vi "ExportDependencyItemRuleContent.vi"(8 "error in (no error)":errorcluster, 10 "IDependencyItemRule in":refnum<class "IDependencyItemRule.lvclass">, 11 "CGrapherDGML in":refnum<class "CGrapherDGML.lvclass">) -> (0 "error out":errorcluster, 1 "Links":T1, 2 "Nodes":T1, 3 "CGrapherDGML":refnum<class "CGrapherDGML.lvclass">)   [LabVIEW 2020, in "DefaultExtensions.lvlib" / "CGrapherDGML.lvclass"]
uses:
  CGrapherDGML.lvclass
  obj/Addons/LabVIEWObjectInterfaces.lvlibp/LabVIEWObjectInterfaces/IDependencyItemRule/IDependencyItemRule.lvclass
  E:/Repos/LVDependencyInspector/obj/Addons/LabVIEWObjectInterfaces.lvlibp/LabVIEWObjectInterfaces/ILabVIEWItem/ILabVIEWItem.lvclass
  obj/Addons/LabVIEWItem.lvlibp/LabVIEWItem/CLabVIEWItem/ConnectionSet.ctl
  CGrapherDGML.lvclass/CGrapherDGML.ctl
  84b6f64b-e02b-4565-8a95-97306d3fff3e.vi
  5ae37459-432d-44eb-8d2b-a2ae9b2d80af.vi
  0dec89c7-531e-457a-9eb0-0c91c63ee5dd.vi
  obj/Addons/LabVIEWItem.lvlibp/LabVIEWItem/CLabVIEWItem/CLabVIEWItem.lvclass
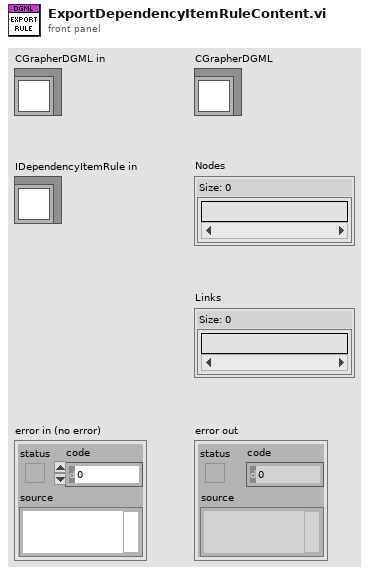
[diagram p1: front panel]
types:
  T1 = typedef "LabVIEWItem.lvlibp/CLabVIEWItem.lvclass/ConnectionSet.ctl" = set{string}
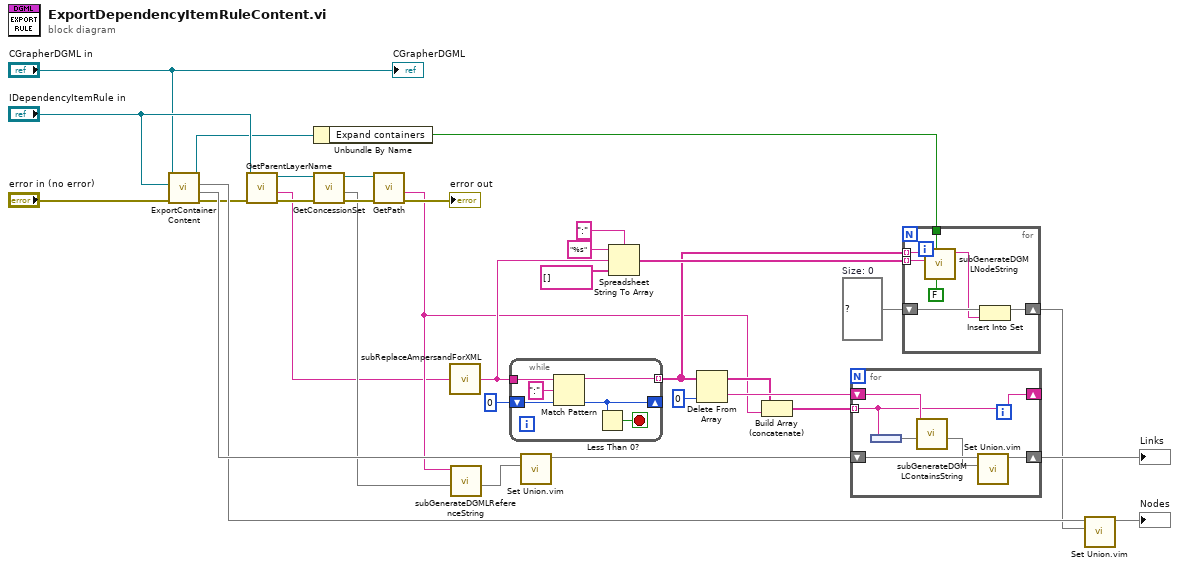
[diagram p0: block diagram]
diagram:
  w20 = set{string} {}  # Size: 0
  n1 = call-dynamic "ExportContainerContent.vi"("error in (no error)"="error in (no error)", "ILabVIEWItem in"="IDependencyItemRule in", "CGrapherDGML in"="CGrapherDGML in") -> ("error out"=w8:errorcluster, "Links"=w31:T1, "Nodes"=w19:T1, "CGrapherDGML"=w1:refnum<class "CGrapherDGML.lvclass">)  [unwired: 5 in]
  n2 = call-dynamic "GetParentLayerName.vi"("error in (no error)"=w8, "IDependencyItemRule in"="IDependencyItemRule in") -> ("error out"=w6:errorcluster, "Parent layer name"=w5:string, "IDependencyItemRule out"=w7:refnum<class "IDependencyItemRule.lvclass">)  [unwired: 7 in]
  n3 = Unbundle By Name(w1) -> ("Expand containers"=w2:bool)
  n4 = call-dynamic "GetConcessionSet.vi"("error in (no error)"=w6, "IDependencyItemRule in"=w7) -> ("error out"=w10:errorcluster, "Concessions"=w9:set{string}, "IDependencyItemRule out"=w11:refnum<class "IDependencyItemRule.lvclass">)  [unwired: 7 in]
  n5 = call-dynamic "GetPath.vi"("error in (no error)"=w10, "ILabVIEWItem in"=w11) -> ("error out"=→"error out":errorcluster, "Path"=w12:string)  [unwired: 7 in, 1 out]
  n6 = call "subReplaceAmpersandForXML.vi"("String"=w5) -> ("result string"=w25:string)
  n7 = call "subGenerateDGMLReferenceString.vi"("References"=w9, "Source"=w12) -> ("Links"=w27:T1)  [unwired: 9 in]
  n8 = while {
    tunnel: w25 -> [w39]
    shift-right: [w37] -> _
    shift-left: 0 ("offset past match") -> [w36]
    tunnel: [w34] -> w15 mode=indexing
    stop <- w35 stop-if-true
    n9 = Match Pattern(string=w39, regular expression=":" ("delimiter (Tab)"), offset (0)=w36) -> (before substring=w34:string, offset past match=w37:i32)  [unwired: 2 out]
    n10 = Less Than 0?(x=w37) -> (x < 0?=w35:bool)
  }
  n11 = call "Set Union.vim"("set 2"=w27, "set 1"=w31) -> ("union"=w26:T1)  [unwired: 9 in]
  n12 = Spreadsheet String To Array(delimiter (Tab)=":", format string="%s", spreadsheet string=w25, array type (2D Dbl)=string[] []) -> (array=w16:string[])
  n13 = Delete From Array(array=w15, index=0) -> (deleted portion=w28:string, array with subset deleted=w14:string[])  [unwired: 1 in]
  n14 = Build Array (concatenate)(w14, w12) -> (w13:string[])
  n15 = for {
    shift-right: [w44] -> _
    shift-left: w28 -> [w45]
    tunnel: w13 -> [w44] mode=indexing
    shift-right: [w40] -> w21
    shift-left: w26 -> [w42]
    n16 = node(w44) -> (w43:set{string})
    n17 = call "subGenerateDGMLContainsString.vi"("Contained"=w43, "Source"=w45) -> ("Links"=w41:T1)  [unwired: 9 in]
    n18 = call "Set Union.vim"("set 2"=w41, "set 1"=w42) -> ("union"=w40:T1)  [unwired: 9 in]
  }
  "Links" <- w21
  n19 = for {
    tunnel: w16 -> [w52] mode=indexing
    tunnel: w15 -> [w51] mode=indexing
    shift-right: [w49] -> w17
    shift-left: w20 -> [w50]
    tunnel: w2 -> [w46]
    n20 = call "subGenerateDGMLNodeString.vi"("Container empty?"=FALSE, "Expand?"=w46, "Label"=w52, "Id"=w51) -> ("Node string"=w48:string)  [unwired: 7 in]
    n21 = Insert Into Set(10:w48, 11:w50) -> (3:w49:set{string})  [unwired: 1 out]
  }
  n22 = call "Set Union.vim"("set 2"=w17, "set 1"=w19) -> ("union"=→"Nodes":T1)  [unwired: 9 in]
  "CGrapherDGML" <- "CGrapherDGML in"
